vi "to_xml.vi"(8 "error in":errorcluster, 11 "HSDIO Settings":T1={"Enable HSDIO Pulses"=TRUE, "Resource Name"="PXI1Slot6", "Clock Rate"=20000000.0, "Array of Script Triggers"=[], "Pulse Generation Script"="script script1\n     Generate RedTrap_compress_temp\nend script", "Start Trigger"={"Wait for start trigger?"=FALSE, "source (PFI 0)"="PFI0", "edge (rising)"=12, "description"=""}, "Hardware alignment quantum\n(in samples)"=1, "Inital State"="", "Idle State"="", "Active Channels"="", "Array of Waveforms"=[], "description"=""} {"Hardware alignment quantum\n(in samples)" min=1 step=1; "Array of Script Triggers"."level" items=["High Level"=34, "Low Level"=35]; "Array of Script Triggers"."edge" items=["Rising Edge"=12, "Falling Edge"=13]; "Start Trigger"."edge (rising)" items=["Rising Edge"=12, "Falling Edge"=13]; "Clock Rate" min=0.0 max=200000000.0 format="%.2p"}) -> (0 "error out":errorcluster, 3 "HSDIO settings string":string)   [LabVIEW 2013, in "HSDIO.lvclass"]
doc: "Saves HSDIO settings in the format:\n\n<EnableHSDIOPulses>%b</EnableHSDIOPulses>\n<ResourceName>%s</ResourceName>\n<ClockRate>%f</ClockRate>\n<unitsPerSecond>%f</unitsPerSecond>\n<HardwareAlignmentQuantum units=\"samples\">%u</HardwareAlignmentQuantum>\n<ArrayOfScriptTriggers columns=\"id, source, type, edge, level\">\n<trigger>%s\\t%s\\t%s\\t%s\\t%s</trigger>\n</ArrayOfScriptTriggers>\n<ChannelsControl columns=\"Description, Active?, Idle State\">\n<channel>%s</channel>\n</ChannelsControl>\n<PulseGenerationScript>%s</PulseGenerationScript>\n<DirectoryToLookForWaveformFiles>%s</DirectoryToLookForWaveformFiles>\n<StartTrigger.WaitForStartTrigger>%b</StartTrigger.WaitForStartTrigger>\n<StartTrigger.source>%s</StartTrigger.source>\n<StartTrigger.edge>%s</StartTrigger.edge>\n\nMTL 2013 Jan 1"
uses:
  HSDIO.lvclass
  <instrlib>/niHSDIO/niHSDIO.llb/niHSDIO_ctl Trigger Script - trigID Values (Ring).ctl
  <instrlib>/niHSDIO/niHSDIO.llb/niHSDIO_ctl Trigger DigEdge - Edge Values (Ring).ctl
  <instrlib>/niHSDIO/niHSDIO.llb/niHSDIO_ctl Trigger Source Values (Ring).ctl
  HSDIO_settings.ctl
  <instrlib>/niHSDIO/niHSDIO.llb/niHSDIO_ctl Trigger DigLvl - Level Values (Ring).ctl
  waveform.ctl
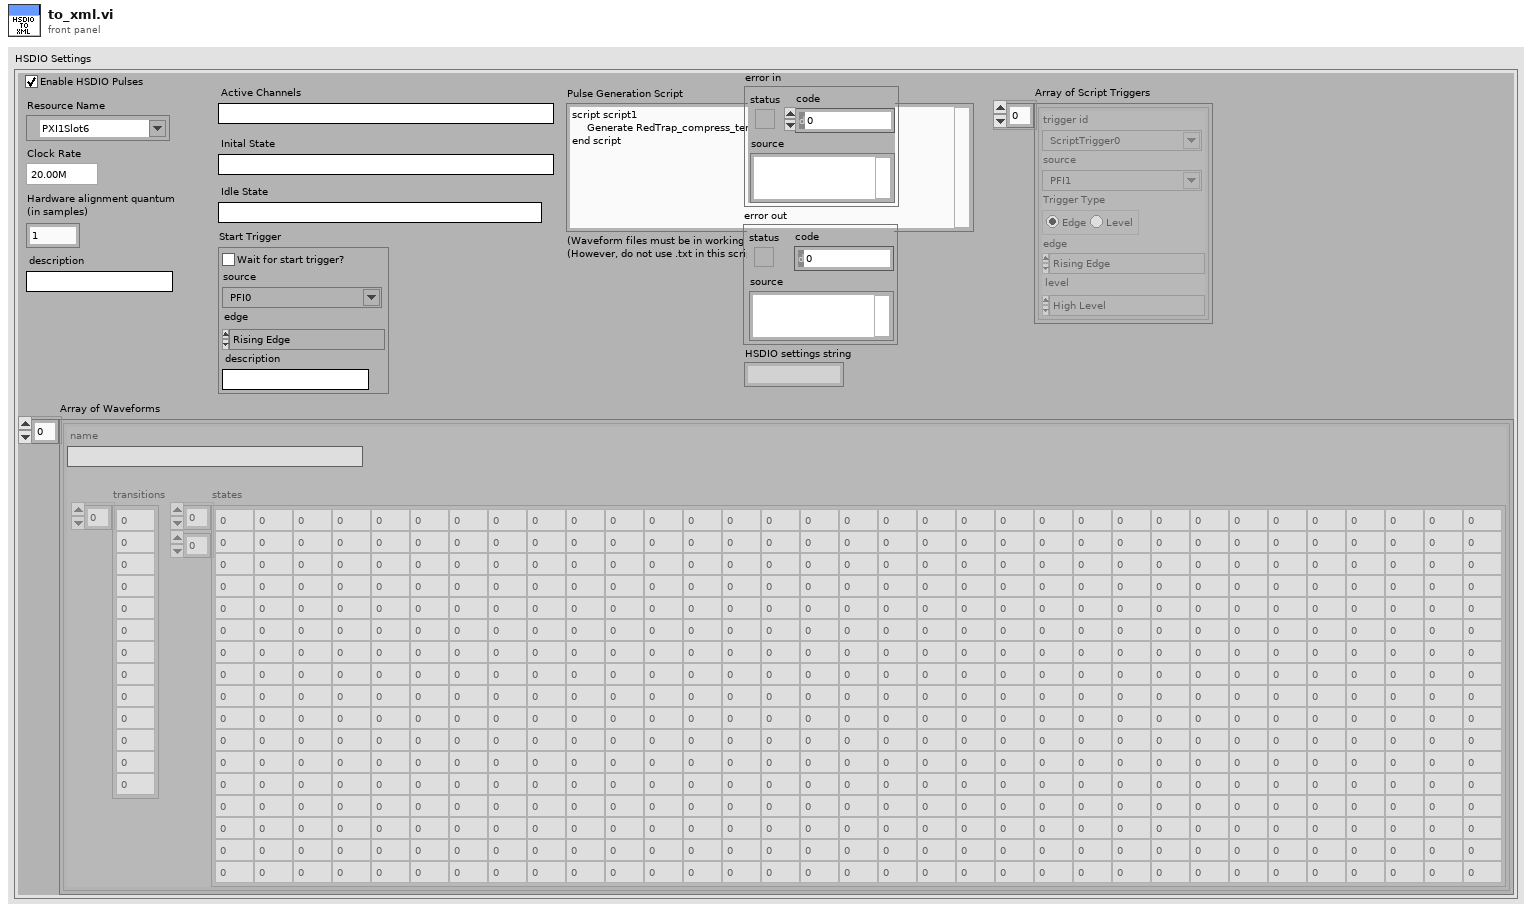
[diagram p1: front panel]
types:
  T1 = typedef "HSDIO.lvclass/HSDIO_settings.ctl" = cluster{"Enable HSDIO Pulses":bool, "Resource Name":refnum<k15>, "Clock Rate":dbl, "Array of Script Triggers":cluster{"trigger id (script trigger 0)":T2, "source (PFI 0)":T3, "Trigger Type":enum32{"Edge", "Level"}, "edge":T4, "level":T5}[], "Pulse Generation Script":string, "Start Trigger":cluster{"Wait for start trigger?":bool, "source (PFI 0)":T3, "edge (rising)":T4, "description":string}, "Hardware alignment quantum\n(in samples)":u16, "Inital State":string, "Idle State":string, "Active Channels":string, "Array of Waveforms":T6[], "description":string}
  T2 = typedef "niHSDIO_ctl Trigger Script - trigID Values (Ring).ctl" = string
  T3 = typedef "niHSDIO_ctl Trigger Source Values (Ring).ctl" = string
  T4 = typedef "niHSDIO_ctl Trigger DigEdge - Edge Values (Ring).ctl" = i32
  T5 = typedef "niHSDIO_ctl Trigger DigLvl - Level Values (Ring).ctl" = i32
  T6 = typedef "HSDIO.lvclass/waveform.ctl" = cluster{"name":string, "transitions":u32[], "states":u8[][]}
  T7 = cluster{"trigger id (script trigger 0)":T2, "source (PFI 0)":T3, "Trigger Type":enum32{"Edge", "Level"}, "edge":T4, "level":T5}[]
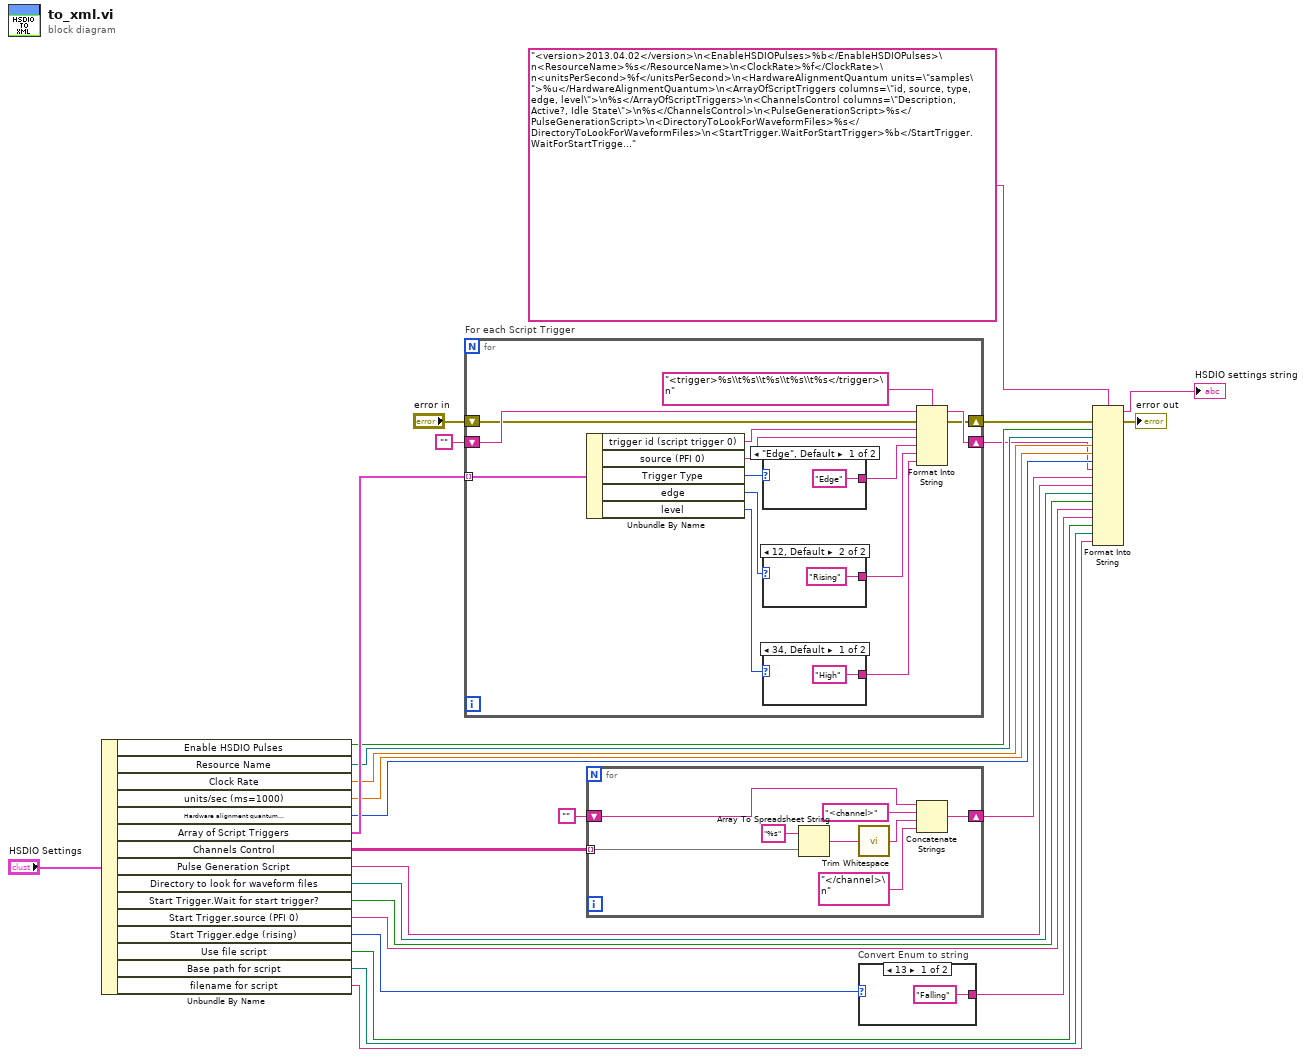
[diagram p0: block diagram]
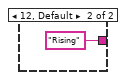
[diagram p2: hidden frame]
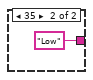
[diagram p3: hidden frame]
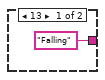
[diagram p4: hidden frame]
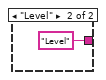
[diagram p5: hidden frame]
diagram:
  n1 = Unbundle By Name("HSDIO Settings") -> ("Enable HSDIO Pulses"=w22:bool, "Resource Name"=w20:refnum<k15>, "Clock Rate"=w19:dbl, "units/sec (ms=1000)"=w18:dbl, "Hardware alignment quantum\n(in samples)"=w17:u16, "Array of Script Triggers"=w24:T7, "Channels Control"=w7:string[][], "Pulse Generation Script"=w15:string, "Directory to look for waveform files"=w14:path, "Start Trigger.Wait for start trigger?"=w13:bool, "Start Trigger.source (PFI 0)"=w12:T3, "Start Trigger.edge (rising)"=w11:T4, "Use file script"=w3:bool, "Base path for script"=w2:path, "filename for script"=w1:string)
  n2 = for "For each Script Trigger" {
    tunnel: w24 -> [w40] mode=indexing
    shift-right: [w34] -> w16
    shift-left: "" -> [w35]
    shift-right: [w32] -> w4
    shift-left: "error in" -> [w33]
    n3 = Unbundle By Name(w40) -> ("trigger id (script trigger 0)"=w39:T2, "source (PFI 0)"=w38:T3, "Trigger Type"=w36:enum32{"Edge", "Level"}, "edge"=w30:T4, "level"=w28:T5)
    n4 = case shown="\"Edge\", Default" w36 {
      tunnel: ["Edge" "Level"] -> w31
      frame "Edge", Default {
      }
      frame "Level" {
      }
    }
    n5 = case shown="12, Default" w30 {
      tunnel: ["Falling" "Rising"] -> w29
      frame 13 {
      }
      frame 12, Default {
      }
    }
    n6 = case shown="34, Default" w28 {
      tunnel: ["High" "Low"] -> w27
      frame 34, Default {
      }
      frame 35 {
      }
    }
    n7 = Format Into String(format string="<trigger>%s\\t%s\\t%s\\t%s\\t%s</trigger>\n", initial string=w35, error in=w33, w39, w38, w31, w29, w27) -> (resulting string=w34:string, error out=w32:errorcluster)
  }
  n8 = for {
    tunnel: w7 -> [w54] mode=indexing
    shift-right: [w49] -> w5
    shift-left: "" -> [w50]
    n9 = Array To Spreadsheet String(array=w54, 3:"%s" ("format string")) -> (spreadsheet string=w48:string)  [unwired: 1 in]
    n10 = call <vilib>:"Trim Whitespace.vi"("string"=w48) -> ("trimmed string"=w47:string)  [unwired: 1 in]
    n11 = Concatenate Strings(w50, "<channel>" ("string"), w47, "</channel>\n" ("string")) -> (w49:string)
  }
  n12 = case "Convert Enum to string" shown="13" w11 {
    tunnel: ["Falling" "Rising"] -> w10
    frame 13 {
    }
    frame 12, Default {
    }
  }
  n13 = Format Into String(format string="<version>2013.04.02</version>\n<EnableHSDIOPulses>%b</EnableHSDIOPulses>\n<ResourceName>%s</ResourceName>\n<ClockRate>%f</ClockRate>\n<unitsPerSecond>%f</unitsPerSecond>\n<HardwareAlignmentQuantum units=\"samples\">%u</HardwareAlignmentQuantum>\n<ArrayOfScriptTriggers columns=\"id, source, type, edge, level\">\n%s</ArrayOfScriptTriggers>\n<ChannelsControl columns=\"Description, Active?, Idle State\">\n%s</ChannelsControl>\n<PulseGenerationScript>%s</PulseGenerationScript>\n<DirectoryToLookForWaveformFiles>%s</DirectoryToLookForWaveformFiles>\n<StartTrigger.WaitForStartTrigger>%b</StartTrigger.WaitForStartTrigger>\n<StartTrigger.source>%s</StartTrigger.source>\n<StartTrigger.edge>%s</StartTrigger.edge>\n<UseFileScript>%b</UseFileScript>\n<BasePathForScript>%s</BasePathForScript>\n<FileNameForScript>%s</FileNameForScript>", error in=w4, w22, w20, w19, w18, w17, w16, w5, w15, w14, w13, w12, w10, w3, w2, w1) -> (resulting string=→"HSDIO settings string":string, error out=→"error out":errorcluster)  [unwired: 1 in]
